vi "Process.vi"(0 "reference in":refnum<class "Logger.lvclass">, 5 "error in":errorcluster) -> (14 "reference out":refnum<class "Logger.lvclass">, 19 "error out":errorcluster)   [LabVIEW 2023, in "Logger.lvclass"]
uses:
  Logger.lvclass
  builds/PowerModuleInterface/PowerModuleInterface.lvlibp/Classes/PowerModule_interface/PowerModuleInterface.lvclass
  Logger.lvclass/Logger.ctl
  <vilib>/Utility/SystemLogging/NI_SystemLogging.lvlib
panel:
  out "error info":errorcluster
  out "Last Command":string
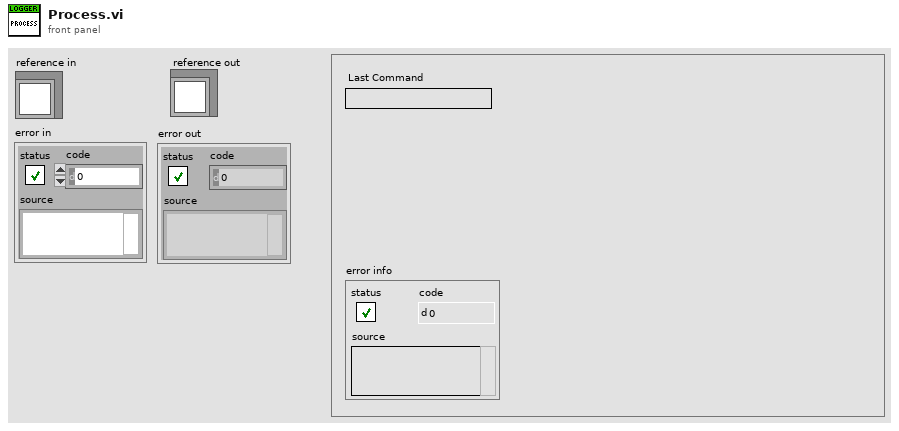
[diagram p1: front panel]
types:
  T1 = cluster{"Core":cluster{"Timeout":i32, "Events":cluster{"EventsToProcess":refnum<event-registration>}, "EventFromProcess":refnum<user-event>, "ProcessSyncQueue":refnum<queue>, "QueueFromProcess":refnum<queue>, "Command":string, "Data":variant}, "Log File Format":string, "Output Directory":path, "Log File Type":enum16{"TDMS", "CSV"}, "TDMS File":refnum<k34>, "CSV File":refnum<file>, "Generated Log":path, "Log Enabled":bool, "Log Created":bool, "Power Module":refnum<class "PowerModuleInterface.lvclass">, "Last Timestamp":dbl}
  T2 = enum16{"open", "open or create", "create or replace", "create", "open (read-only)"}
  T3 = enum16{"open", "replace", "create", "open or create", "replace or create", "replace or create with confirmation"}
  T4 = enum32{"Invalid", "Standard", "Closed", "Hidden", "Minimized", "Maximized"}
  T5 = cluster{"EventsToProcess":refnum<event-registration>}
  T6 = typedef "Logger.lvclass/ObjectAttributes.ctl" = cluster{"Output Directory":path, "Log File Type":enum16{"TDMS", "CSV"}, "Power Module":refnum<class "PowerModuleInterface.lvclass">}
  T7 = typedef "PowerModuleInterface.lvlibp/PowerModuleInterface.lvclass/Measurements.ctl" = cluster{"measured voltage (V)":dbl, "measured current (A)":dbl, "setpoint voltage (V)":dbl, "setpoint current (A)":dbl, "timestamp":dbl}
  T8 = typedef "NI_BC_client.lvlib/MStream_grpc_CyclerMeasurement.ctl" = cluster{"measured_voltage":sgl, "measured_current":sgl, "setpoint_voltage":sgl, "setpoint_current":sgl, "timestamp":i64}
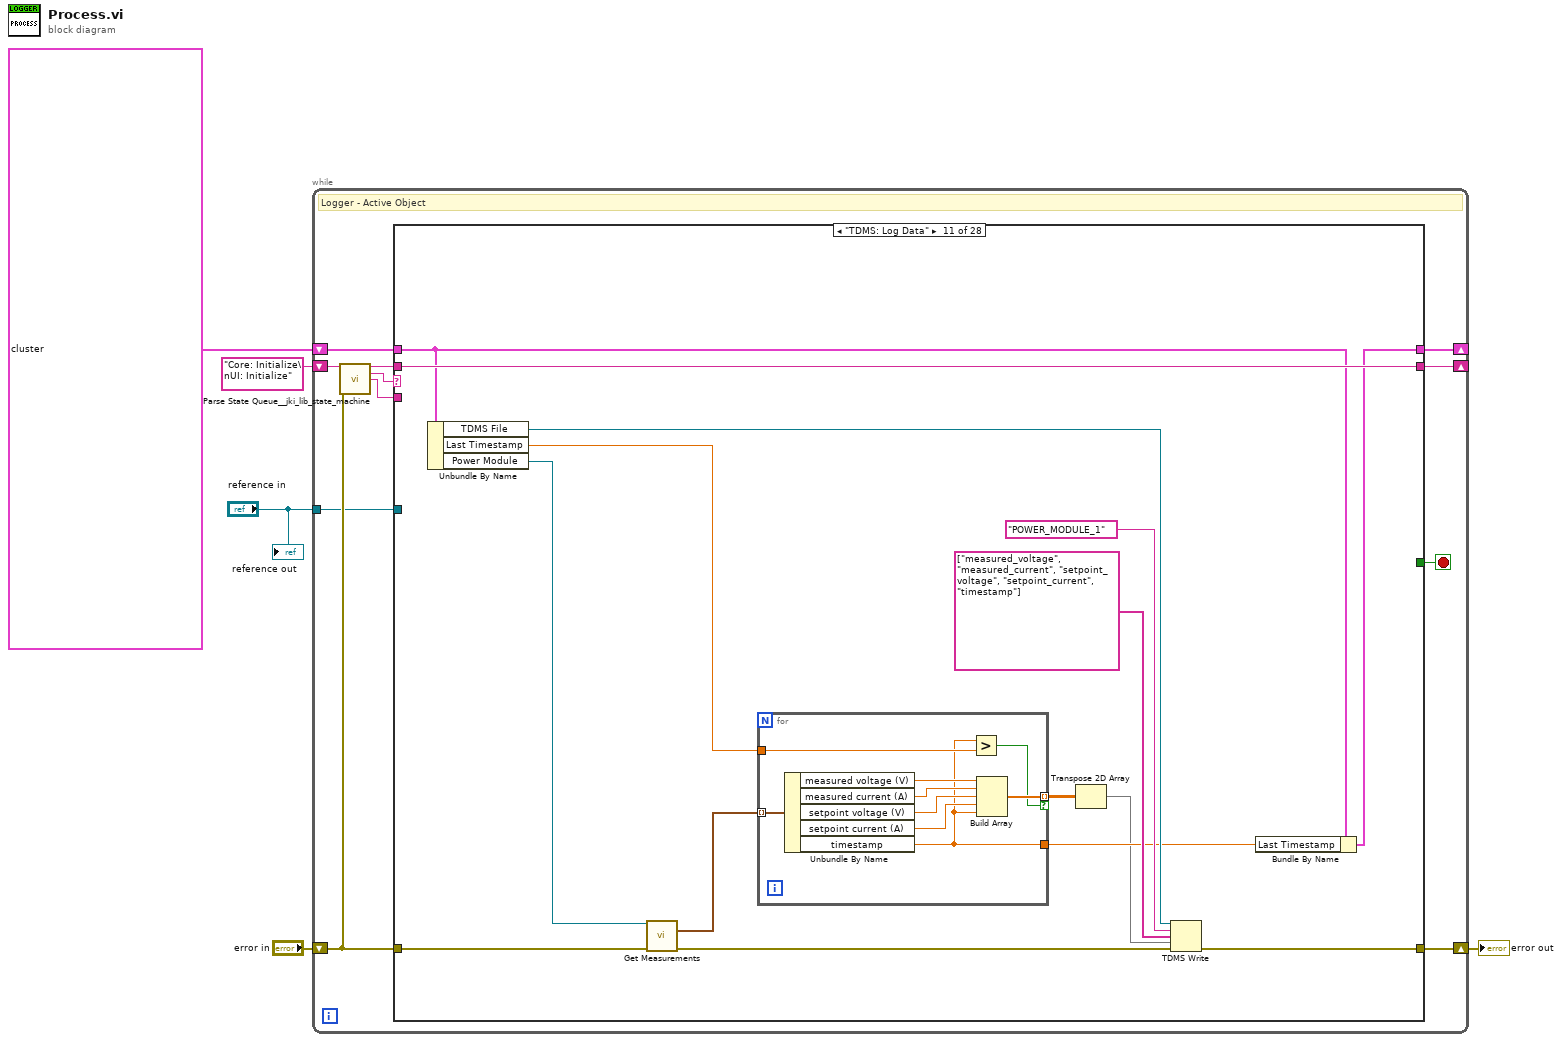
[diagram p0: block diagram]
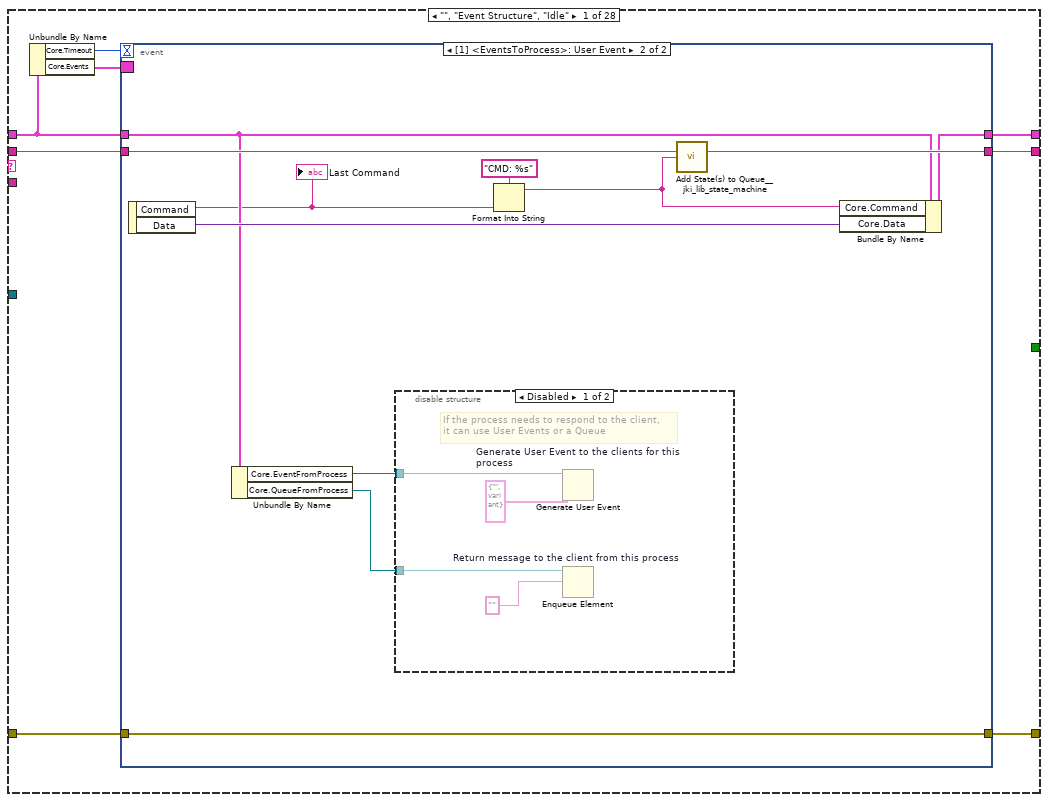
[diagram p2: hidden frame]
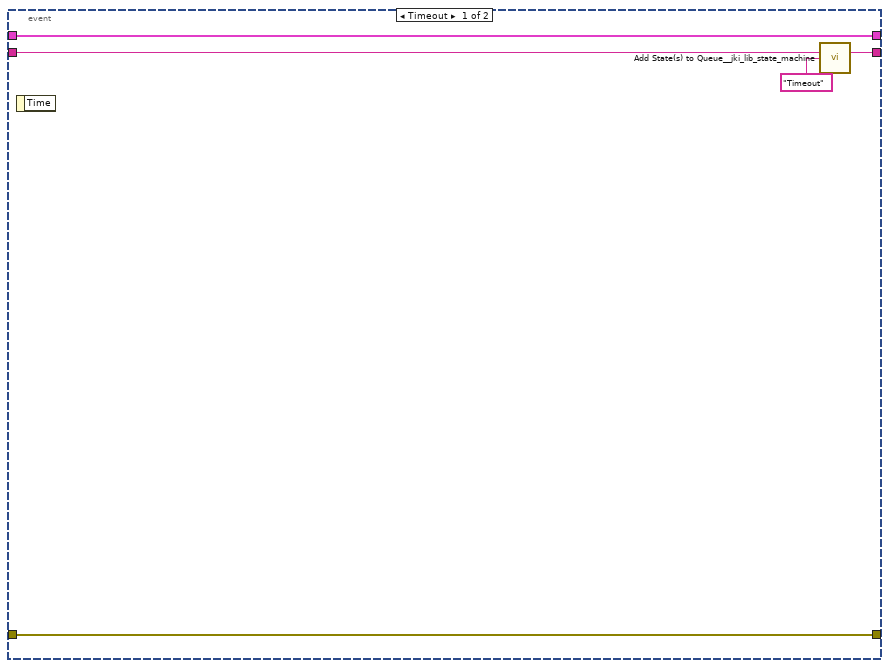
[diagram p3: hidden frame]
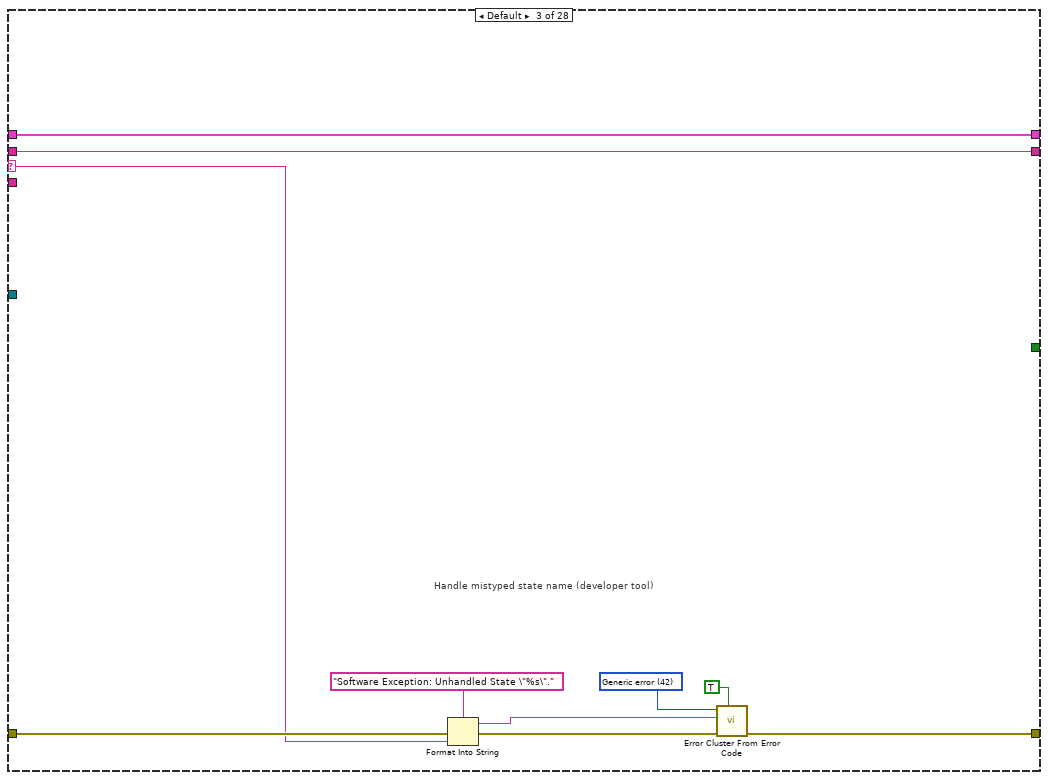
[diagram p6: hidden frame]
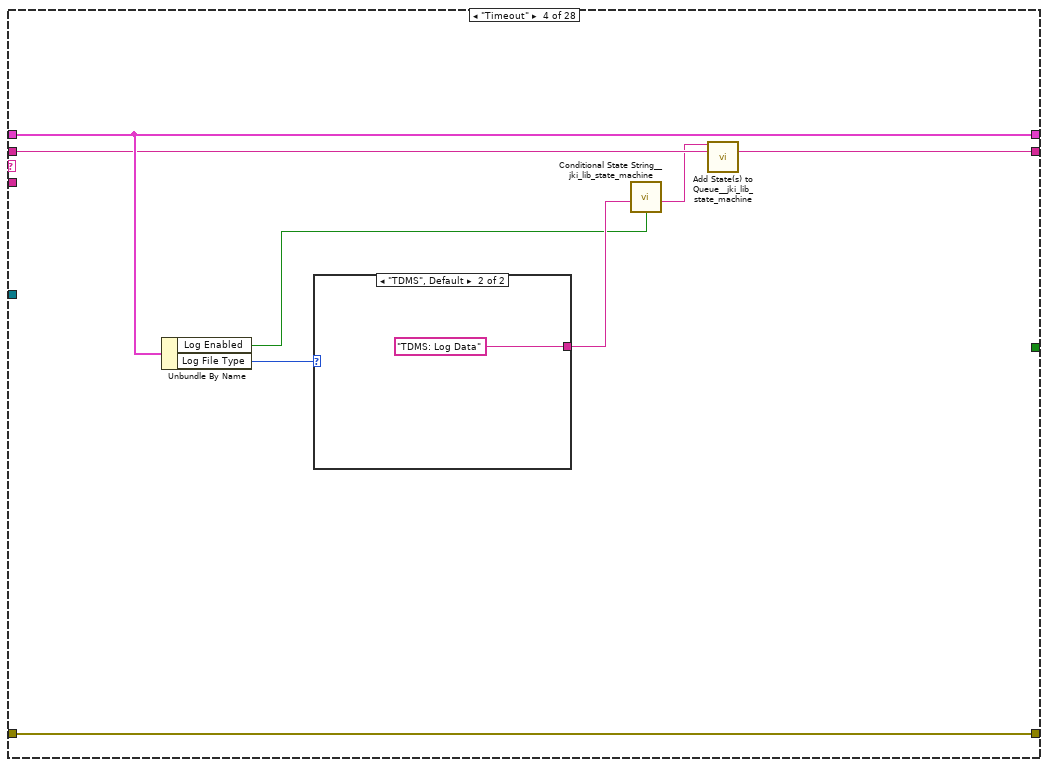
[diagram p7: hidden frame]
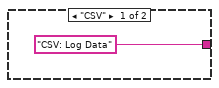
[diagram p8: hidden frame]
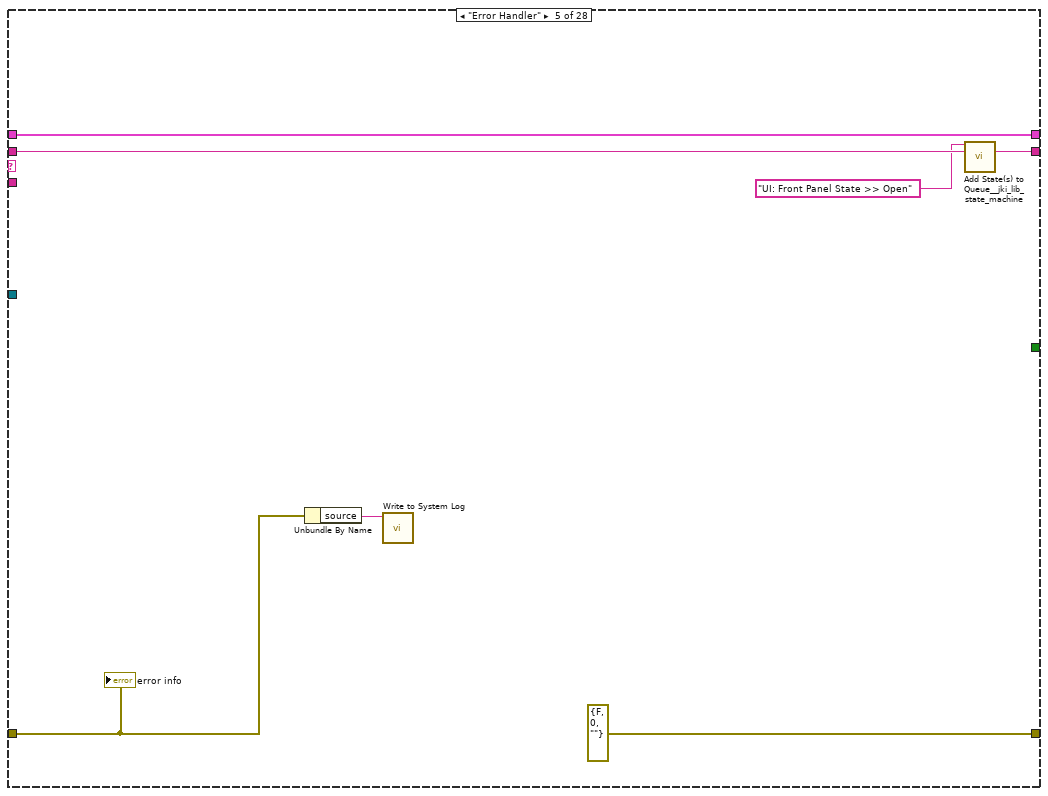
[diagram p9: hidden frame]
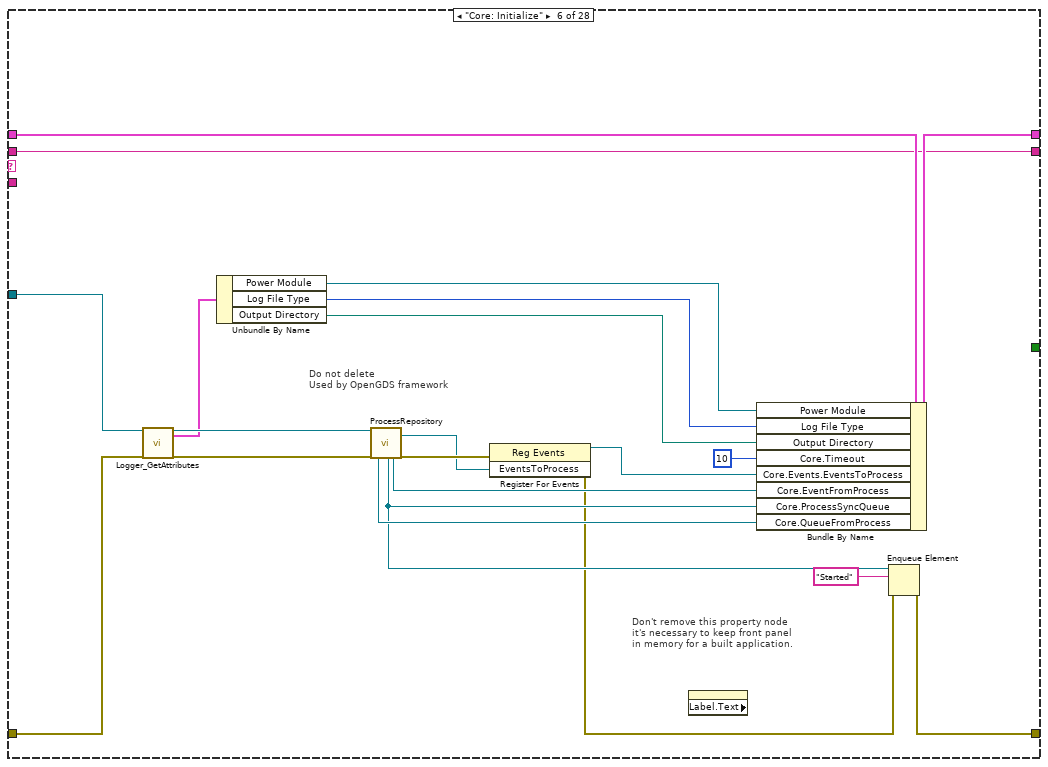
[diagram p10: hidden frame]
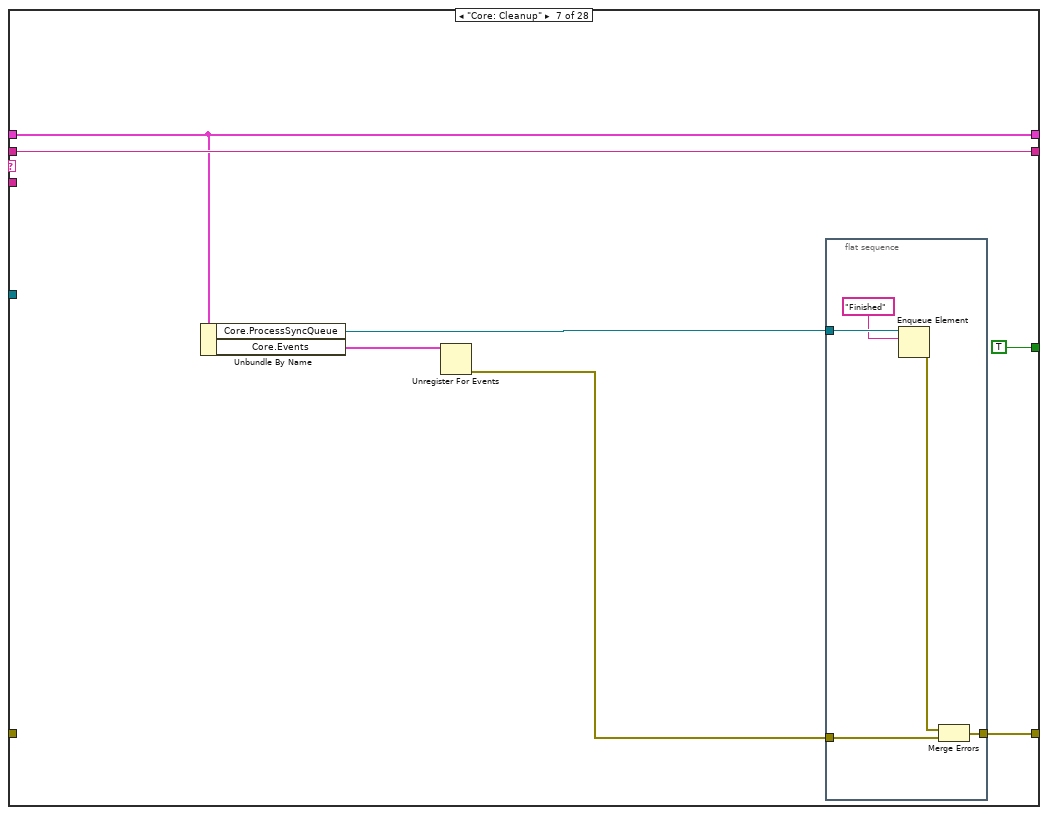
[diagram p11: hidden frame]
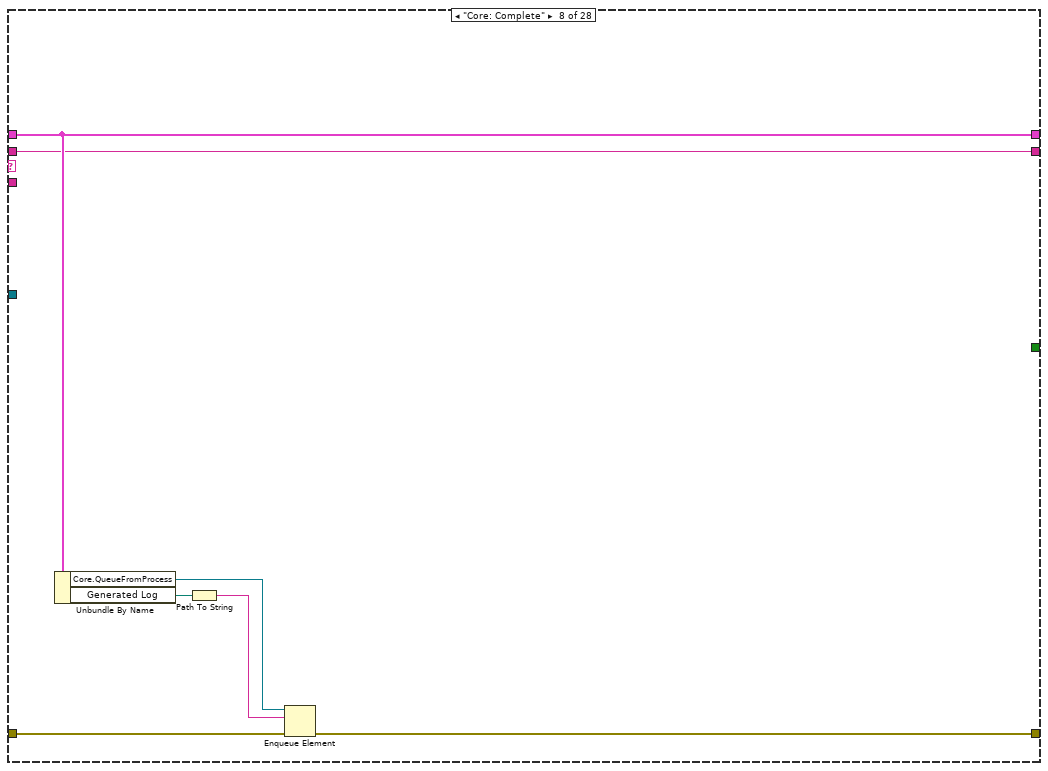
[diagram p12: hidden frame]
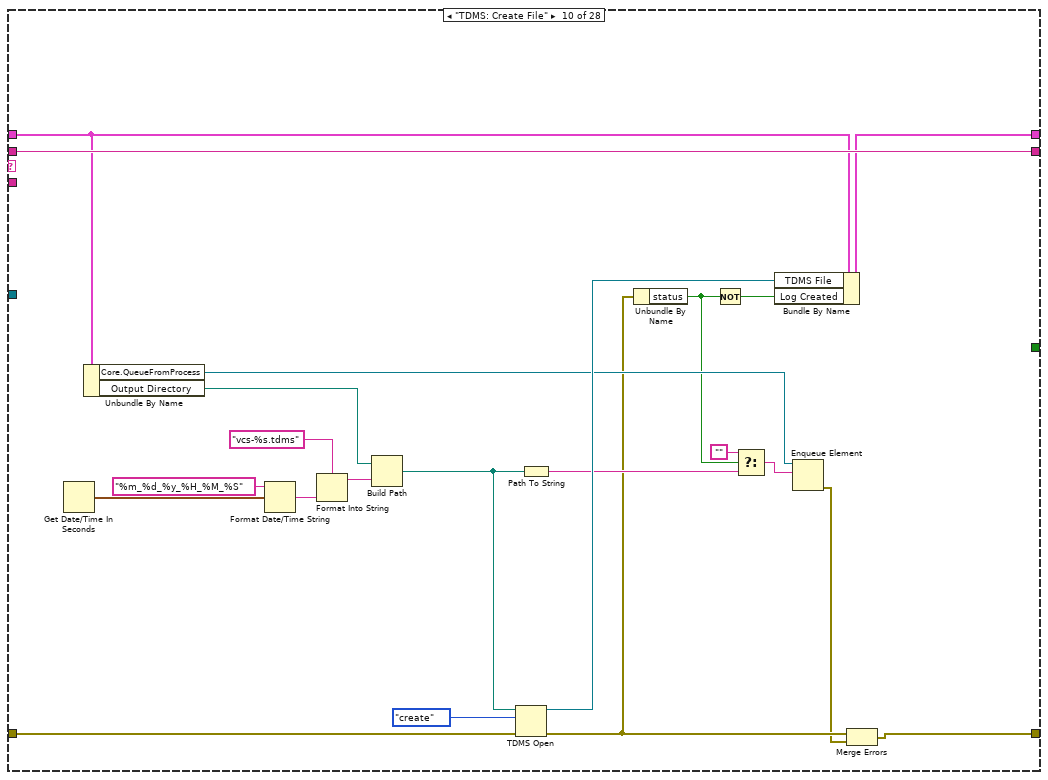
[diagram p14: hidden frame]
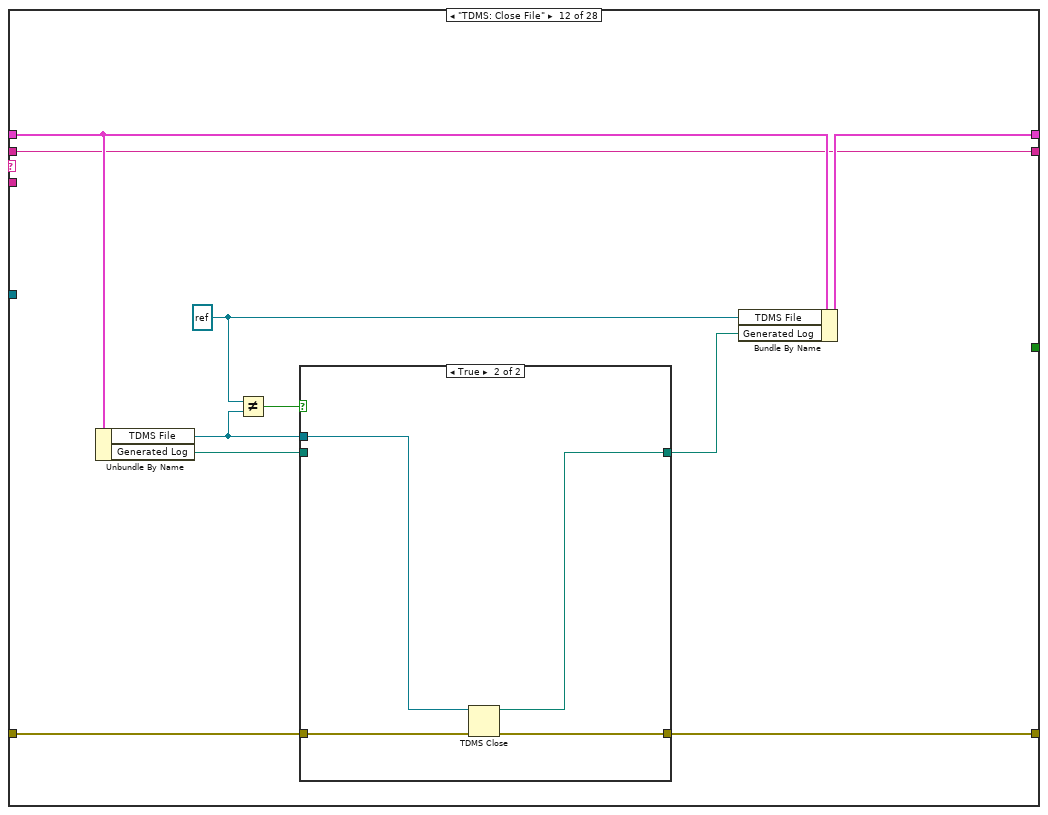
[diagram p15: hidden frame]
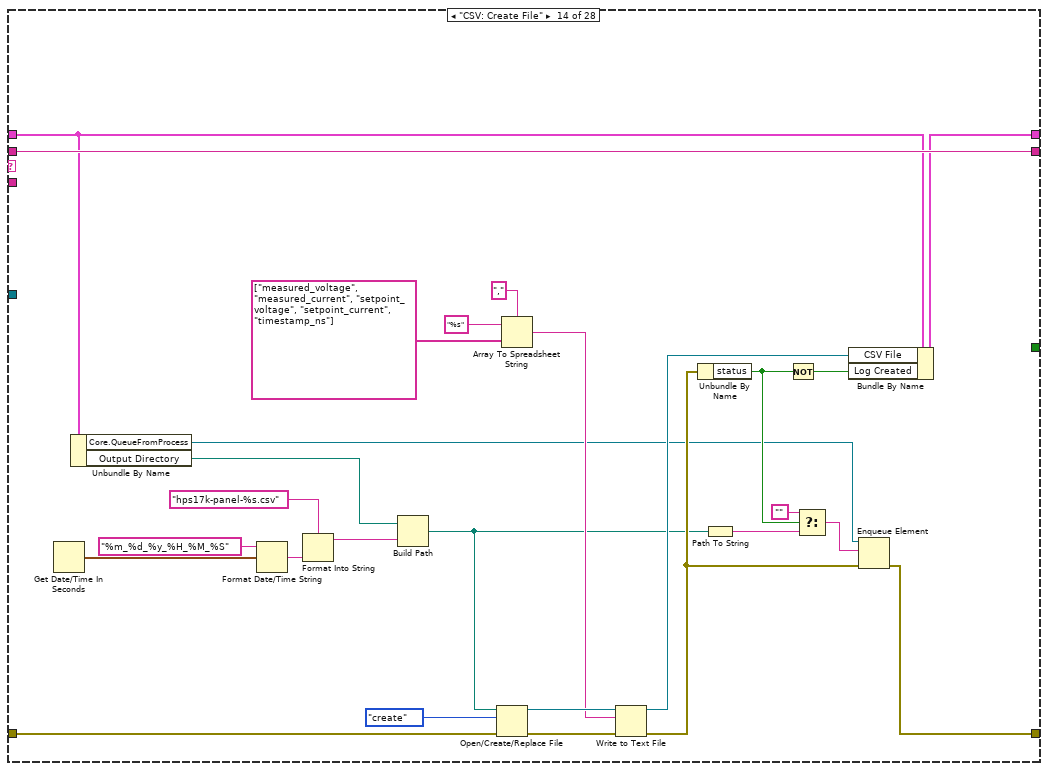
[diagram p18: hidden frame]
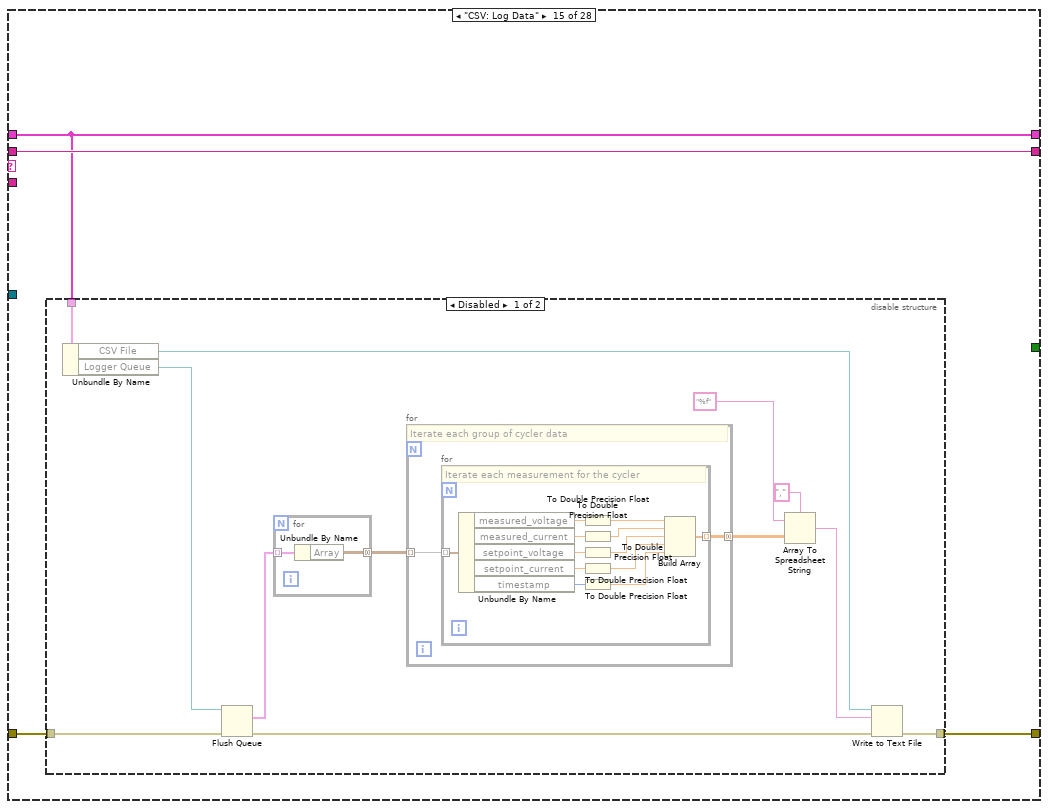
[diagram p19: hidden frame]
diagram:
  n1 = while {
    shift-right: [w15] -> w4
    shift-left: "error in" -> [w16]
    shift-right: [w8] -> _
    shift-left: "Core: Initialize\nUI: Initialize" ("States Out") -> [w11]
    shift-right: [w14] -> _
    shift-left: T1 {"Core"={"Timeout"=-1, "Events"={"EventsToProcess"=refnum}, "EventFromProcess"=refnum, "ProcessSyncQueue"=refnum, "QueueFromProcess"=refnum, "Command"="", "Data"=variant}, "Log File Format"="", "Output Directory"=path "", "Log File Type"=enum."TDMS", "TDMS File"=refnum, "CSV File"=refnum, "Generated Log"=path "", "Log Enabled"=FALSE, "Log Created"=FALSE, "Power Module"=refnum, "Last Timestamp"=0.0} ("LocalVariables") -> [w13]
    tunnel: "reference in" -> [w6]
    stop <- w7 stop-if-true
    # "Logger - Active Object"
    n2 = call <vilib>:"Parse State Queue__jki_lib_state_machine.vi"("State Queue"=w11, "Error In (no error)"=w16) -> ("Remaining States"=w10:string, "Current State"=w12:string, "Arguments"=w9:string)  [unwired: 11 in]
    n3 = case shown="\"TDMS: Log Data\"" w12 {
      selector: w12 -> [_ _ w48 _ _ _ _ _ _ _ _ _ _ _ _ _ _ _ _ _ _ _ _ _ _ _ _ _]
      tunnel: w16 -> [w18 w47 w50 w65 w70 w81 _ w112 w117 w138 w147 w171 w182 w202 w211 w249 w253 w254 w277 _ w284 w290 w300 w308 w317 w318 w329 w332]
      tunnel: [w19 w47 w49 w65 errorcluster {"status"=FALSE, "code"=0, "source"=""} ("error constant") w95 w98 w111 w117 w118 w153 w170 w182 w190 w210 w248 w253 w254 w277 w278 w284 w290 w300 w308 w317 w318 w329 w331] -> w15
      tunnel: [w24 w46 w57 w64 w74 w94 w99 w114 w116 w136 w142 w173 w181 w199 w212 w246 w252 w256 w269 w279 w283 w289 w299 w304 w316 w323 w325 w336] -> w14
      tunnel: w13 -> [w20 w46 w57 w64 w74 w93 w99 w114 w116 w134 w144 w172 w181 w200 w212 w247 w252 w256 w269 w279 w283 w289 w299 w304 w316 w322 w326 w335]
      tunnel: w10 -> [w22 w45 w56 w62 w73 w76 w102 w110 w115 w139 w154 w164 w180 w209 w213 w243 w251 w257 w276 w281 w282 _ w296 w306 w315 w324 w328 w337]
      tunnel: w9 -> [_ _ _ _ _ _ _ _ _ _ _ _ _ _ _ _ _ w255 _ _ _ _ _ _ w312 _ _ _]
      tunnel: [w21 w45 w56 w61 w72 w76 w102 w110 w115 w139 w154 w164 w180 w209 w213 w243 w251 w257 w276 w281 w282 w286 w297 w305 w314 w324 w328 w337] -> w8
      tunnel: [_ _ _ _ _ _ TRUE _ _ _ _ _ _ _ _ _ _ _ _ _ _ _ _ _ _ _ _ _] -> w7
      tunnel: w6 -> [_ _ _ _ _ w84 _ _ _ _ _ _ _ _ _ _ _ _ _ _ _ _ _ _ _ _ _ _]
      frame "", "Event Structure", "Idle" {
        n4 = Unbundle By Name(w20) -> ("Core.Timeout"=w17:i32, "Core.Events"=w23:T5)
        n5 = event shown="[1] <EventsToProcess>: User Event" {
          selector: w23 -> [_ _]
          dyn-events: _ -> [_ _]
          timeout: w17 -> [_ _]
          tunnel: w20 -> [w29 w33]
          tunnel: [w29 w38] -> w24
          tunnel: [w27 w40] -> w21
          tunnel: w22 -> [w28 w39]
          tunnel: [w25 w34] -> w19
          tunnel: w18 -> [w25 w34]
          event Timeout {
            n6 = event-data() -> ()  [unwired: 1 in, 1 out]
            n7 = call <vilib>:"Add State(s) to Queue__jki_lib_state_machine.vi"("State(s) in (\"\")"=w28, "State(s) at Back (\"\")"="Timeout" ("State(s) at Back (\"\")")) -> ("States Out"=w27:string)  [unwired: 13 in]
          }
          event User Event {
            n8 = event-data() -> ("Command"=w31:string, "Data"=w37:variant)  [unwired: 1 in]
            "Last Command" <- w31
            n9 = Unbundle By Name(w33) -> ("Core.EventFromProcess"=w36:refnum<user-event>, "Core.QueueFromProcess"=w35:refnum<queue>)
            n10 = disable-structure shown="Disabled" {
              disable-tunnel: w36 -> [w44 _]
              disable-tunnel: w35 -> [w43 _]
              frame Disabled {
                # "If the process needs to respond to the client,\nit can use User Events or a Queue"
                n11 = Generate User Event "Generate User Event to the clients for this process"(user event=w44, event data cluster=cluster{"Command":string, "Data":variant} {"Command"="", "Data"=variant} ("event data")) -> ()  [unwired: 2 in, 2 out]
                n12 = Enqueue Element "Return message to the client from this process"(queue=w43, element="") -> ()  [unwired: 2 in, 3 out]
              }
              frame Enabled {
              }
            }
            n13 = Format Into String(format string="CMD: %s", w31) -> (resulting string=w30:string)  [unwired: 2 in, 1 out]
            n14 = call <vilib>:"Add State(s) to Queue__jki_lib_state_machine.vi"("State(s) in (\"\")"=w39, "State(s) at Back (\"\")"=w30) -> ("States Out"=w40:string)  [unwired: 13 in]
            n15 = Bundle By Name(cluster=w33, "Core.Command"=w30, "Core.Data"=w37) -> (w38:T1)
          }
        }
      }
      frame "---------- Core ----------" {
      }
      frame Default {
        w54 = 42 items=["No error", "Argument error", "Memory is full", "Out of zone", "End of file", "File already open", "Generic file I/O error", "File not found", "File permission error", "Disk is full", "Duplicate path", "Too many files open", "System feature not enabled", "Resource file not found", "Cannot add resource", "Resource not found", "Image not found", "Image memory error", "Pen does not exist", "Config type invalid", "Config token not found", "Config parse error", "Config memory error", "Bad external code format", "Bad external code offset", "External code not present", "Null window", "Destroy window error", "Null menu", "Print aborted", "Bad print record", "Print driver error", "Windows error during printing", "Memory error during printing", "Print dialog error", "Generic print error", "Invalid device refnum", "Device not found", "Device parameter error", "Device unit error", "Cannot open device", "Device call aborted", "Generic error", "Cancelled by user", "Object ID too low", "Object ID too high", "Object not in heap", "Unknown heap", "Unknown object (invalid DefProc)", "Unknown object (DefProc not in table)", "Message out of range", "Invalid (null) method", "Unknown message", "Manager call not supported", "Bad address", "Network operation in progress", "Network operation timed out", "Connection is busy", "Network attribute not supported", "Network error", "Address in use", "System out of memory", "Connection aborted", "Connection refused", "Not connected", "Already connected", "Connection closed", "Initialization error (interapplication manager)", "Bad occurrence", "Wait on unbound occurrence handler", "Occurrence queue overflow", "Datalog type conflict", "Unused", "Unrecognized type (interapplication manager)", "Memory corrupt", "Failed to make temporary DLL", "Old CIN version", "Drag socket not found", "Failed to load drop-object", "Failed to register OLE object", "Failed to release OLE object", "Format specifier type mismatch", "Unknown format specifier", "Too few format specifiers", "Too many format specifiers", "Scan failed", "Newer CIN version", "Error converting to variant", "Runtime menu error", "Password tampered", "Variant attribute not found", "Incompatible variant data type", "Event data is not available", "Event Store is not present", "Occurrence is not found", "Event Queue is not created", "Event info is not available", "Refnum passed is NULL", "Error retrieving Class GUID", "Error retrieving CoClass GUID", "Error retrieving TypeLib GUID.", "Bad built application magic bytes.", "Specific driver is different from the specific driver associated with the Logical Name.", "There is no session opened to the class driver.", "Max Error", "MAX - Error with config objects", "MAX - Error loading configuration", "MAX - Group not supported"]
        # "Handle mistyped state name (developer tool)"
        n16 = Format Into String(format string="Software Exception: Unhandled State \"%s\"." ("message"), error in=w50, w48) -> (resulting string=w53:string, error out=w52:errorcluster)  [unwired: 1 in]
        n17 = call <vilib>:"Error Cluster From Error Code.vi"("show call chain? (False)"=TRUE, "error in (no error)"=w52, "error message (\"\")"=w53, "error code (0)"=w54) -> ("error out"=w49:errorcluster)  [unwired: 5 in]
      }
      frame "Timeout" {
        n18 = Unbundle By Name(w64) -> ("Log Enabled"=w58:bool, "Log File Type"=w63:enum16{"TDMS", "CSV"})
        n19 = case shown="\"TDMS\", Default" w63 {
          tunnel: ["CSV: Log Data" ("States Out") "TDMS: Log Data" ("States Out")] -> w60
          frame "CSV" {
          }
          frame "TDMS", Default {
          }
        }
        n20 = call <vilib>:"Conditional State String__jki_lib_state_machine.vi"("Do State(s)?"=w58, "State"=w60) -> ("State Out"=w59:string)  [unwired: 7 in]
        n21 = call <vilib>:"Add State(s) to Queue__jki_lib_state_machine.vi"("State(s) in Front (\"\")"=w59, "State(s) in (\"\")"=w62) -> ("States Out"=w61:string)  [unwired: 13 in]
      }
      frame "Error Handler" {
        n22 = Unbundle By Name(w70) -> ("source"=w68:string)
        n23 = call <vilib>:"Write to System Log.vi"("message"=w68) -> ()  [unwired: 10 in, 1 out]
        n24 = call <vilib>:"Add State(s) to Queue__jki_lib_state_machine.vi"("State(s) in Front (\"\")"="UI: Front Panel State >> Open" ("State(s) at Back (\"\")"), "State(s) in (\"\")"=w73) -> ("States Out"=w72:string)  [unwired: 13 in]
        "error info" <- w70
      }
      frame "Core: Initialize" {
        # "Do not delete\nUsed by OpenGDS framework"
        # "Don't remove this property node\nit's necessary to keep front panel\nin memory for a built application."
        # "Template created by VI Technologies"
        n25 = call "Logger_GetAttributes.vi"("reference in"=w84, "Error In"=w81) -> ("reference out"=w83:refnum<class "Logger.lvclass">, "Data"=w80:T6, "Error Out"=w82:errorcluster)  [unwired: 14 in, 1 out]
        n26 = Unbundle By Name(w80) -> ("Power Module"=w75:refnum<class "PowerModuleInterface.lvclass">, "Log File Type"=w78:enum16{"TDMS", "CSV"}, "Output Directory"=w79:path)
        n27 = call "ProcessRepository.vi"("reference in"=w83, "Error In"=w82) -> ("QueueFromProcess"=w88:refnum<queue>, "ProcessSyncQueue"=w86:refnum<queue>, "EventFromProcess"=w89:refnum<user-event>, "EventsToProcess"=w91:refnum<user-event>, "Error Out"=w92:errorcluster)  [unwired: 10 in, 3 out]
        n28 = register-events(error in=w92, w91) -> (reference out=w90:refnum<event-registration>, error out=w85:errorcluster)  [unwired: 1 in]
        n29 = property on="reference in" class="LVClassControl (strict)" props=["Label", "Text"]() -> ()  [unwired: 2 in, 3 out]
        n30 = Bundle By Name(cluster=w93, "Power Module"=w75, "Log File Type"=w78, "Output Directory"=w79, "Core.Timeout"=10, "Core.Events.EventsToProcess"=w90, "Core.EventFromProcess"=w89, "Core.ProcessSyncQueue"=w86, "Core.QueueFromProcess"=w88) -> (w94:T1)
        n31 = Enqueue Element(queue=w86, element="Started", error in (no error)=w85) -> (error out=w95:errorcluster)  [unwired: 1 in, 2 out]
      }
      frame "Core: Cleanup" {
        n32 = Unbundle By Name(w99) -> ("Core.ProcessSyncQueue"=w100:refnum<queue>, "Core.Events"=w97:T5)
        n33 = Unregister For Events(event registration refnum=w97) -> (error out=w96:errorcluster)  [unwired: 1 in]
        n34 = flat-sequence {
          tunnel: [w106] -> w98
          tunnel: w100 -> [w105]
          tunnel: w96 -> [w104]
          frame #0 {
            n35 = Enqueue Element(queue=w105, element="Finished") -> (error out=w107:errorcluster)  [unwired: 2 in, 2 out]
            n36 = Merge Errors(w107, w104) -> (w106:errorcluster)
          }
        }
      }
      frame "Core: Complete" {
        n37 = Unbundle By Name(w114) -> ("Core.QueueFromProcess"=w113:refnum<queue>, "Generated Log"=w109:path)
        n38 = Path To String(path=w109) -> (string=w108:string)
        n39 = Enqueue Element ("Return message to the client from this process")(queue=w113, element=w108, error in (no error)=w112) -> (error out=w111:errorcluster)  [unwired: 1 in, 2 out]
      }
      frame "---------- TDMS ----------" {
      }
      frame "TDMS: Create File" {
        n40 = Get Date/Time In Seconds() -> (seconds since 1Jan1904=w130:timestamp)
        n41 = Unbundle By Name(w134) -> ("Core.QueueFromProcess"=w125:refnum<queue>, "Output Directory"=w132:path)
        n42 = Format Date/Time String(time format string (%c)="%m_%d_%y_%H_%M_%S", seconds (now)=w130) -> (date/time string=w129:string)  [unwired: 1 in]
        n43 = Format Into String(format string="vcs-%s.tdms", w129) -> (resulting string=w131:string)  [unwired: 2 in, 1 out]
        n44 = Build Path(base path=w132, name or relative path=w131) -> (appended path=w126:path)
        n45 = TDMS Open(8:w138, 10:T2."create" ("operation (0:open)"), 11:w126) -> (0:w120:errorcluster, 3:w135:refnum<k34>)  [unwired: 4 in]
        n46 = Path To String(path=w126) -> (string=w122:string)
        n47 = Unbundle By Name(w120) -> ("status"=w123:bool)
        n48 = Not(x=w123) -> (.not. x?=w127:bool)
        n49 = Select(t="", s=w123, f=w122) -> (s? t:f=w121:string)
        n50 = Bundle By Name(cluster=w134, "TDMS File"=w135, "Log Created"=w127) -> (w136:T1)
        n51 = Enqueue Element(queue=w125, element=w121) -> (error out=w119:errorcluster)  [unwired: 2 in, 2 out]
        n52 = Merge Errors(w120, w119) -> (w118:errorcluster)
      }
      frame "TDMS: Log Data" {
        n53 = Unbundle By Name(w144) -> ("TDMS File"=w152:refnum<k34>, "Last Timestamp"=w145:dbl, "Power Module"=w146:refnum<class "PowerModuleInterface.lvclass">)
        n54 = call-dynamic "Get Measurements.vi"("object in"=w146, "Error In"=w147) -> ("measurements"=w148:T7[], "Error Out"=w149:errorcluster)  [unwired: 11 in, 1 out]
        n55 = for {
          tunnel: [w163] -> w141 mode=indexing if=w156
          tunnel: w148 -> [w162] mode=indexing
          tunnel: w145 -> [w157]
          tunnel: [w155] -> w143
          n56 = Unbundle By Name(w162) -> ("measured voltage (V)"=w161:dbl, "measured current (A)"=w160:dbl, "setpoint voltage (V)"=w159:dbl, "setpoint current (A)"=w158:dbl, "timestamp"=w155:dbl)
          n57 = Greater?(x=w155, y=w157) -> (0:w156:bool)
          n58 = Build Array(w161, w160, w159, w158, w155) -> (w163:dbl[])
        }
        n59 = Transpose 2D Array(2D array=w141) -> (transposed array=w140:dbl[][])
        n60 = TDMS Write(0:w152, 5:"POWER_MODULE_1" ("group name in (Untitled)"), 7:string[] ["measured_voltage", "measured_current", "setpoint_voltage", "setpoint_current", "timestamp"] ("channel name(s) in (Untitled)"), 9:w140, 11:w149) -> (15:w153:errorcluster)  [unwired: 1 in, 3 out]
        n61 = Bundle By Name(cluster=w144, "Last Timestamp"=w143) -> (w142:T1)
      }
      frame "TDMS: Close File" {
        w168 = refnum<k34> refnum ("TDMS File")
        n62 = Unbundle By Name(w172) -> ("TDMS File"=w169:refnum<k34>, "Generated Log"=w166:path)
        n63 = Not Equal?(x=w168, y=w169) -> (x != y?=w167:bool)
        n64 = case shown="True" w167 {
          tunnel: w171 -> [w175 w179]
          tunnel: [w175 w178] -> w170
          tunnel: w169 -> [_ w177]
          tunnel: w166 -> [w174 _]
          tunnel: [w174 w176] -> w165
          frame False {
          }
          frame True {
            n65 = TDMS Close(8:w179, 11:w177) -> (0:w178:errorcluster, 3:w176:path)
          }
        }
        n66 = Bundle By Name(cluster=w172, "TDMS File"=w168, "Generated Log"=w165) -> (w173:T1)
      }
      frame "---------- CSV ----------" {
      }
      frame "CSV: Create File" {
        n67 = Get Date/Time In Seconds() -> (seconds since 1Jan1904=w206:timestamp)
        n68 = Unbundle By Name(w200) -> ("Core.QueueFromProcess"=w184:refnum<queue>, "Output Directory"=w203:path)
        n69 = Format Date/Time String(time format string (%c)="%m_%d_%y_%H_%M_%S", seconds (now)=w206) -> (date/time string=w205:string)  [unwired: 1 in]
        n70 = Format Into String(format string="hps17k-panel-%s.csv", w205) -> (resulting string=w207:string)  [unwired: 2 in, 1 out]
        n71 = Build Path(base path=w203, name or relative path=w207) -> (appended path=w188:path)
        n72 = Open/Create/Replace File(file path (use dialog)=w188, error in=w202, operation (0:open)=T3."create") -> (refnum out=w198:refnum<file>, error out=w197:errorcluster)  [unwired: 3 in, 1 out]
        n73 = Array To Spreadsheet String(delimiter (Tab)=",", array=string[] ["measured_voltage", "measured_current", "setpoint_voltage", "setpoint_current", "timestamp_ns"] ("channel name(s) in (Untitled)"), 3:"%s" ("format string")) -> (spreadsheet string=w193:string)
        n74 = Write to Text File(file (use dialog)=w198, text=w193, error in=w197) -> (refnum out=w189:refnum<file>, error out=w191:errorcluster)  [unwired: 1 in, 1 out]
        n75 = Unbundle By Name(w191) -> ("status"=w186:bool)
        n76 = Path To String(path=w188) -> (string=w187:string)
        n77 = Not(x=w186) -> (.not. x?=w192:bool)
        n78 = Select(t="", s=w186, f=w187) -> (s? t:f=w185:string)
        n79 = Bundle By Name(cluster=w200, "CSV File"=w189, "Log Created"=w192) -> (w199:T1)
        n80 = Enqueue Element(queue=w184, element=w185, error in (no error)=w191) -> (error out=w190:errorcluster)  [unwired: 1 in, 2 out]
      }
      frame "CSV: Log Data" {
        n81 = disable-structure shown="Disabled" {
          disable-tunnel: w212 -> [w225 _]
          disable-tunnel: w211 -> [w224 w242]
          disable-tunnel: [w221 w242] -> w210
          frame Disabled {
            n82 = Unbundle By Name(w225) -> ("CSV File"=w220:refnum<file>, "Logger Queue"=w223:refnum<queue>)
            n83 = Flush Queue(queue=w223, error in (no error)=w224) -> (remaining elements=w216:cluster{"Array":T8[][]}[], error out=w222:errorcluster)  [unwired: 1 out]
            n84 = for {
              tunnel: w216 -> [w241] mode=indexing
              tunnel: [w240] -> w215 mode=concatenating
              n85 = Unbundle By Name(w241) -> ("Array"=w240:T8[][])
            }
            n86 = for {
              tunnel: w215 -> [w227] mode=indexing
              tunnel: [w226] -> w214 mode=concatenating
              # "Iterate each group of cycler data"
              n87 = for {
                tunnel: w227 -> [w239] mode=indexing
                tunnel: [w238] -> w226 mode=indexing
                # "Iterate each measurement for the cycler"
                n88 = Unbundle By Name(w239) -> ("measured_voltage"=w237:sgl, "measured_current"=w236:sgl, "setpoint_voltage"=w235:sgl, "setpoint_current"=w234:sgl, "timestamp"=w233:i64)
                n89 = To Double Precision Float(number=w237) -> (double precision float=w232:dbl)
                n90 = To Double Precision Float(number=w236) -> (double precision float=w231:dbl)
                n91 = To Double Precision Float(number=w235) -> (double precision float=w230:dbl)
                n92 = To Double Precision Float(number=w234) -> (double precision float=w229:dbl)
                n93 = To Double Precision Float(number=w233) -> (double precision float=w228:dbl)
                n94 = Build Array(w232, w231, w230, w229, w228) -> (w238:dbl[])
              }
            }
            n95 = Array To Spreadsheet String(delimiter (Tab)=",", array=w214, 3:"%f" ("format string")) -> (spreadsheet string=w217:string)
            n96 = Write to Text File(file (use dialog)=w220, text=w217, error in=w222) -> (error out=w221:errorcluster)  [unwired: 1 in, 2 out]
          }
          frame Enabled {
          }
        }
      }
      frame "CSV: Close File" {
        n97 = Unbundle By Name(w247) -> ("CSV File"=w250:refnum<file>)
        n98 = Close File(refnum=w250, error in=w249) -> (path=w244:path, error out=w248:errorcluster)
        n99 = Bundle By Name(cluster=w247, "CSV File"=refnum<file> refnum, "Generated Log"=w244) -> (w246:T1)
      }
      frame "---------- UI ----------" {
      }
      frame "UI: Front Panel State" {
        n100 = case shown="\"Close\"" w255 {
          frame "Open", Default {
            n101 = property class="VI"() -> ("FP.State"=w258:T4)  [unwired: 2 in, 2 out]
            n102 = case shown="Default" w258 {
              frame Default {
                n103 = invoke class="VI" method="FP.Open"("Activate"=TRUE, "State"=T4."Standard") -> ()  [unwired: 3 in, 5 out]
              }
              frame "Standard" {
              }
            }
          }
          frame "Close" {
            n104 = property class="VI"() -> ("FP.State"=w261:T4)  [unwired: 2 in, 2 out]
            n105 = case shown="Default" w261 {
              frame "Closed" {
              }
              frame Default {
                n106 = invoke class="VI" method="FP.Close"() -> ()  [unwired: 3 in, 3 out]
              }
            }
          }
        }
      }
      frame "UI: Initialize" {
        n107 = property class="VI"() -> ("Name"=w275:string)  [unwired: 2 in, 2 out]
        n108 = Match Pattern(string=w275, regular expression="\\2Evi$") -> (before substring=w273:string)  [unwired: 1 in, 3 out]
        n109 = Reverse String(1:w273) -> (0:w272:string)
        n110 = Match Pattern(string=w272, regular expression=":") -> (before substring=w270:string, after substring=w268:string)  [unwired: 1 in, 2 out]
        n111 = Match Pattern(string=w268, regular expression="\\2E") -> (after substring=w266:string)  [unwired: 1 in, 3 out]
        n112 = Reverse String(1:w266) -> (0:w265:string)
        n113 = Reverse String(1:w270) -> (0:w264:string)
        n114 = Format Into String(format string="%s %s", w265, w264) -> (resulting string=w263:string)  [unwired: 2 in, 1 out]
        n115 = property class="VI"("Front Panel.Title"=w263) -> ()  [unwired: 2 in, 2 out]
      }
      frame "UI: Cleanup" {
        n116 = property class="VI"() -> (error out=w278:errorcluster, "FP.State"=w280:T4)  [unwired: 2 in, 1 out]
        n117 = case shown="\"Standard\", Default" w280 {
          frame "Closed" {
          }
          frame "Standard", Default {
            n118 = invoke class="VI" method="FP.Close"() -> ()  [unwired: 3 in, 3 out]
          }
        }
      }
      frame "---------- CMD ----------" {
      }
      frame "CMD: Exit" {
        n119 = Unbundle By Name(w289) -> ("Log File Type"=w288:enum16{"TDMS", "CSV"})
        n120 = case shown="\"TDMS\", Default" w288 {
          tunnel: ["TDMS: Close File" ("State(s) in Front (\"\")") "CSV: Close File" ("State(s) in Front (\"\")")] -> w285
          frame "TDMS", Default {
          }
          frame "CSV" {
          }
        }
        n121 = call <vilib>:"Add State(s) to Queue__jki_lib_state_machine.vi"("State(s) in Front (\"\")"=w285, "State(s) in (\"\")"="UI: Cleanup\nCore: Cleanup" ("State(s) at Back (\"\")")) -> ("States Out"=w286:string)  [unwired: 13 in]
      }
      frame "CMD: Close Log" {
        n122 = Unbundle By Name(w299) -> ("Log File Type"=w298:enum16{"TDMS", "CSV"})
        n123 = case shown="\"CSV\"" w298 {
          tunnel: ["TDMS: Close File" ("State(s) in Front (\"\")") "CSV: Close File" ("State(s) in Front (\"\")")] -> w295
          frame "TDMS", Default {
          }
          frame "CSV" {
          }
        }
        n124 = call <vilib>:"Add State(s) to Queue__jki_lib_state_machine.vi"("State(s) in (\"\")"=w295, "State(s) at Back (\"\")"="Core: Complete" ("State(s) at Back (\"\")")) -> ("States Out"=w294:string)  [unwired: 13 in]
        n125 = call <vilib>:"Add State(s) to Queue__jki_lib_state_machine.vi"("State(s) in Front (\"\")"=w294, "State(s) in (\"\")"=w296) -> ("States Out"=w297:string)  [unwired: 13 in]
      }
      frame "CMD: Create Log" {
        n126 = Unbundle By Name(w304) -> ("Log File Type"=w303:enum16{"TDMS", "CSV"})
        n127 = case shown="\"TDMS\", Default" w303 {
          tunnel: ["TDMS: Create File" ("States Out") "CSV: Create File" ("States Out")] -> w307
          frame "TDMS", Default {
          }
          frame "CSV" {
          }
        }
        n128 = call <vilib>:"Add State(s) to Queue__jki_lib_state_machine.vi"("State(s) in Front (\"\")"=w307, "State(s) in (\"\")"=w306) -> ("States Out"=w305:string)  [unwired: 13 in]
      }
      frame "CMD: Front Panel State" {
        n129 = Format Into String(format string="UI: Front Panel State>>%s" ("string"), w312) -> (resulting string=w311:string)  [unwired: 2 in, 1 out]
        n130 = call <vilib>:"Add State(s) to Queue__jki_lib_state_machine.vi"("State(s) in (\"\")"=w315, "State(s) at Back (\"\")"=w311) -> ("States Out"=w314:string)  [unwired: 13 in]
      }
      frame "CMD: Start Log" {
        n131 = Unbundle By Name(w322) -> ("Log Created"=w320:bool)
        n132 = And(x=TRUE ("Enable"), y=w320) -> (x .and. y?=w319:bool)
        n133 = Bundle By Name(cluster=w322, "Log Enabled"=w319) -> (w323:T1)
      }
      frame "CMD: Stop Log" {
        n134 = Bundle By Name(cluster=w326, "Log Enabled"=FALSE ("Enable")) -> (w325:T1)
      }
      frame "CMD: Update Directory" {
        n135 = Unbundle By Name(w335) -> ("Output Directory"=w334:path, "Core.Data"=w333:variant)
        n136 = Variant To Data(error in=w332, type=w334, Variant=w333) -> (data=w330:path, error out=w331:errorcluster)
        n137 = Bundle By Name(cluster=w335, "Output Directory"=w330) -> (w336:T1)
      }
    }
  }
  "error out" <- w4
  "reference out" <- "reference in"
